vi "ExecPratAula01.vi"() -> ()   [LabVIEW 2020]
panel:
  out "Meter":dbl(knob) scale=0.0..100.0
  in  "N Value":fxp<+/-,64,32>
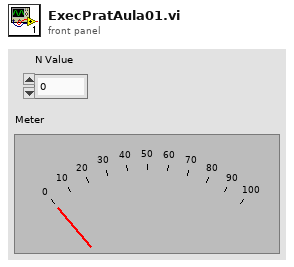
[diagram p1: front panel]
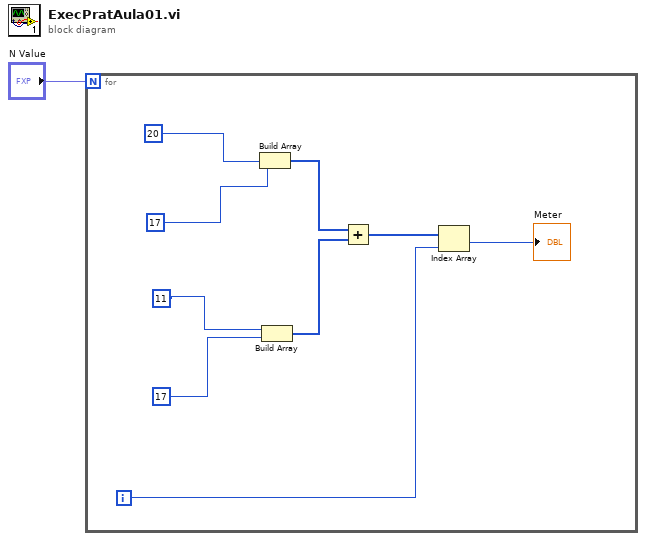
[diagram p0: block diagram]
diagram:
  n1 = for {
    N: "N Value" -> [_]
    i -> [w7]
    n2 = Build Array(20, 17) -> (w10:i32[])
    n3 = Build Array(11, 17) -> (w9:i32[])
    n4 = Add(x=w10, y=w9) -> (x+y=w8:i32[])
    n5 = Index Array(array=w8, index=w7) -> (element=→"Meter":i32)
  }
